vi "_Get Panel Bounds.vi"(1 "Panel Height":i16=300, 2 "Panel Width":i16=600, 3 "Zero-based Panel #":i32) -> (0 "PanelBounds":T1)   [LabVIEW 2012]
doc: "_Get Panelbounds.vi\n\nPurpose: VI output, the cluster \"Panelbounds\", specifies the left, top, right & bottom for a panel., to tile multiple windows of a specified width across a screen of any screen resolution.\n\nThe \"Windowbounds\" property really should be the property being calculated and set. However during initial coding, any attempt to dynamically change the \"Windowbounds\" property resulted in a crash. For whatever reason, the was not the case when the \"Panelbounds\" property is set. The \"Panelbounds\" are calculated taking into account the size of the borders of a window (ie toolbar, edges, etc) so that when the panel is resized, the window appears in a tiled location.\n\nThe other property, 0-based array index, specifies the (tiled) location on-screen that the window will appear. Index 0 will always appear in the upper left corner of the screen. After that, as many windows as possible will be tiled horizontally across the screen. Once a row is filled, subsequently opened windows are placed in the next available row."
panel:
  # "Get Panelbounds"
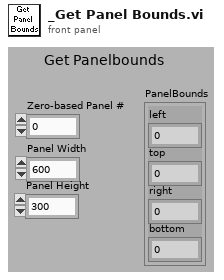
[diagram p1: front panel]
types:
  T1 = cluster{"left":i16, "top":i16, "right":i16, "bottom":i16}
  T2 = typedef "LVRectTypeDef.ctl" = cluster{"Left":i16, "Top":i16, "Right":i16, "Bottom":i16}
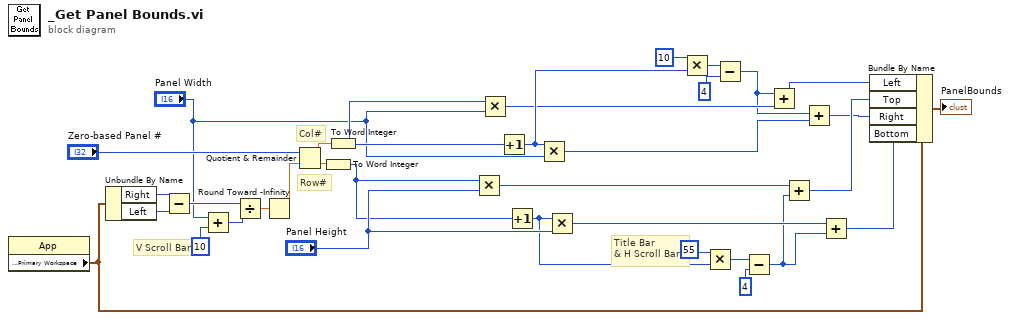
[diagram p0: block diagram]
diagram:
  # "Title Bar\n& H Scroll Bar"
  # "V Scroll Bar"
  # "Col#"
  # "Row#"
  n1 = property class="App"() -> ("Display:Primary Workspace"=w6:T2)  [unwired: 2 in, 2 out]
  n2 = Unbundle By Name(w6) -> ("Right"=w33:i16, "Left"=w34:i16)
  n3 = Subtract(x=w33, y=w34) -> (x-y=w32:i16)
  n4 = Add(x="Panel Width", y=i16 10) -> (x+y=w9:i16)
  n5 = Divide(x=w32, y=w9) -> (x/y=w31:dbl)
  n6 = Round Toward -Infinity(1:w31) -> (0:w30:dbl)
  n7 = Quotient & Remainder(x="Zero-based Panel #", y=w30) -> (x-y*floor(x/y)=w13:dbl, floor(x/y)=w11:dbl)
  n8 = To Word Integer(number=w11) -> (16bit integer=w10:i16)
  n9 = To Word Integer(number=w13) -> (16bit integer=w12:i16)
  n10 = Multiply(x=w10, y="Panel Height") -> (x*y=w20:i16)
  n11 = Multiply(x=w12, y="Panel Width") -> (x*y=w25:i16)
  n12 = Increment(x=w12) -> (x+1=w26:i16)
  n13 = Increment(x=w10) -> (x+1=w22:i16)
  n14 = Multiply(x=w26, y="Panel Width") -> (x*y=w24:i16)
  n15 = Multiply(x=w22, y="Panel Height") -> (x*y=w21:i16)
  n16 = Multiply(x=i16 10, y=w26) -> (x*y=w19:i16)
  n17 = Multiply(x=i16 55, y=w22) -> (x*y=w16:i16)
  n18 = Subtract(x=w19, y=i16 4) -> (x-y=w17:i16)
  n19 = Subtract(x=w16, y=i16 4) -> (x-y=w15:i16)
  n20 = Add(x=w17, y=w25) -> (x+y=w2:i16)
  n21 = Add(x=w20, y=w15) -> (x+y=w3:i16)
  n22 = Add(x=w17, y=w24) -> (x+y=w1:i16)
  n23 = Add(x=w21, y=w15) -> (x+y=w4:i16)
  n24 = Bundle By Name(cluster=w6, "Left"=w2, "Top"=w3, "Right"=w1, "Bottom"=w4) -> (→"PanelBounds":T2)
